vi "MultiChannelMES4HWSyncExample.vi"() -> ()   [LabVIEW 2025]
uses:
  PalmSens/PalmSens.lvclass
  PalmSens/MeasurementsResult.ctl
  PalmSens/MeasurementResults.ctl
  PalmSens/LiveCurveResult.ctl
  C:/Users/stef/code/palmsenssdk/labview/PalmSens/Libraries/PalmSens.Core.Simplified.LabVIEW.dll
  PalmSens/Libraries/PalmSens.Core.Simplified.LabVIEW.dll
panel:
  out "Array 2":string[](array[string])
  out "Is Measuring 2":bool
  in  "PalmSens.lvclass 2":refnum<class "PalmSens.lvclass">
  out "Measurements":T1
  out "MethodSCRIPT":refnum<k24>
  out "Array":string[](array[string])
  out "Is Measuring":bool
  in  "PalmSens.lvclass":refnum<class "PalmSens.lvclass">
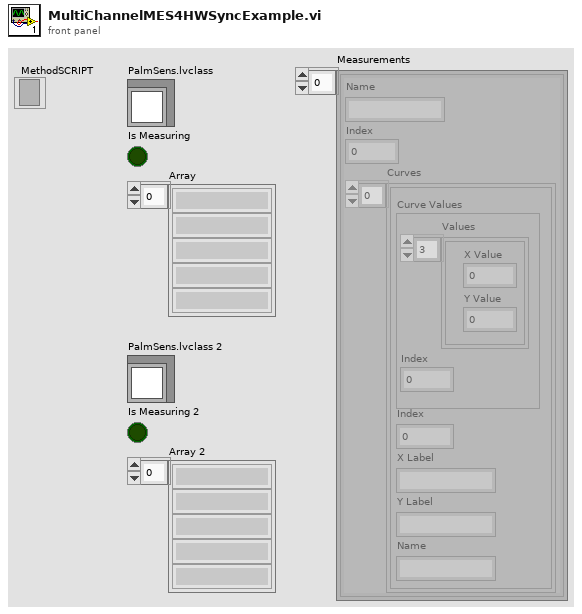
[diagram p1: front panel]
types:
  T1 = typedef "MeasurementsResult.ctl" = cluster{"Name":string, "Curves":T2, "Index":i32}[]
  T2 = typedef "MeasurementResults.ctl" = T3[]
  T3 = typedef "LiveCurveResult.ctl" = cluster{"X Label":string, "Y Label":string, "Name":string, "Index":i16, "Curve Values":cluster{"Values":cluster{"X Value":dbl, "Y Value":dbl}[], "Index":i16}}
  T4 = typedef "ActiveMeasurementInfo.ctl" = cluster{"Active Measurement":refnum<k24>, "Is Measuring Refnum":refnum<vi>, "Live Curve Result Refnum":refnum<vi>}
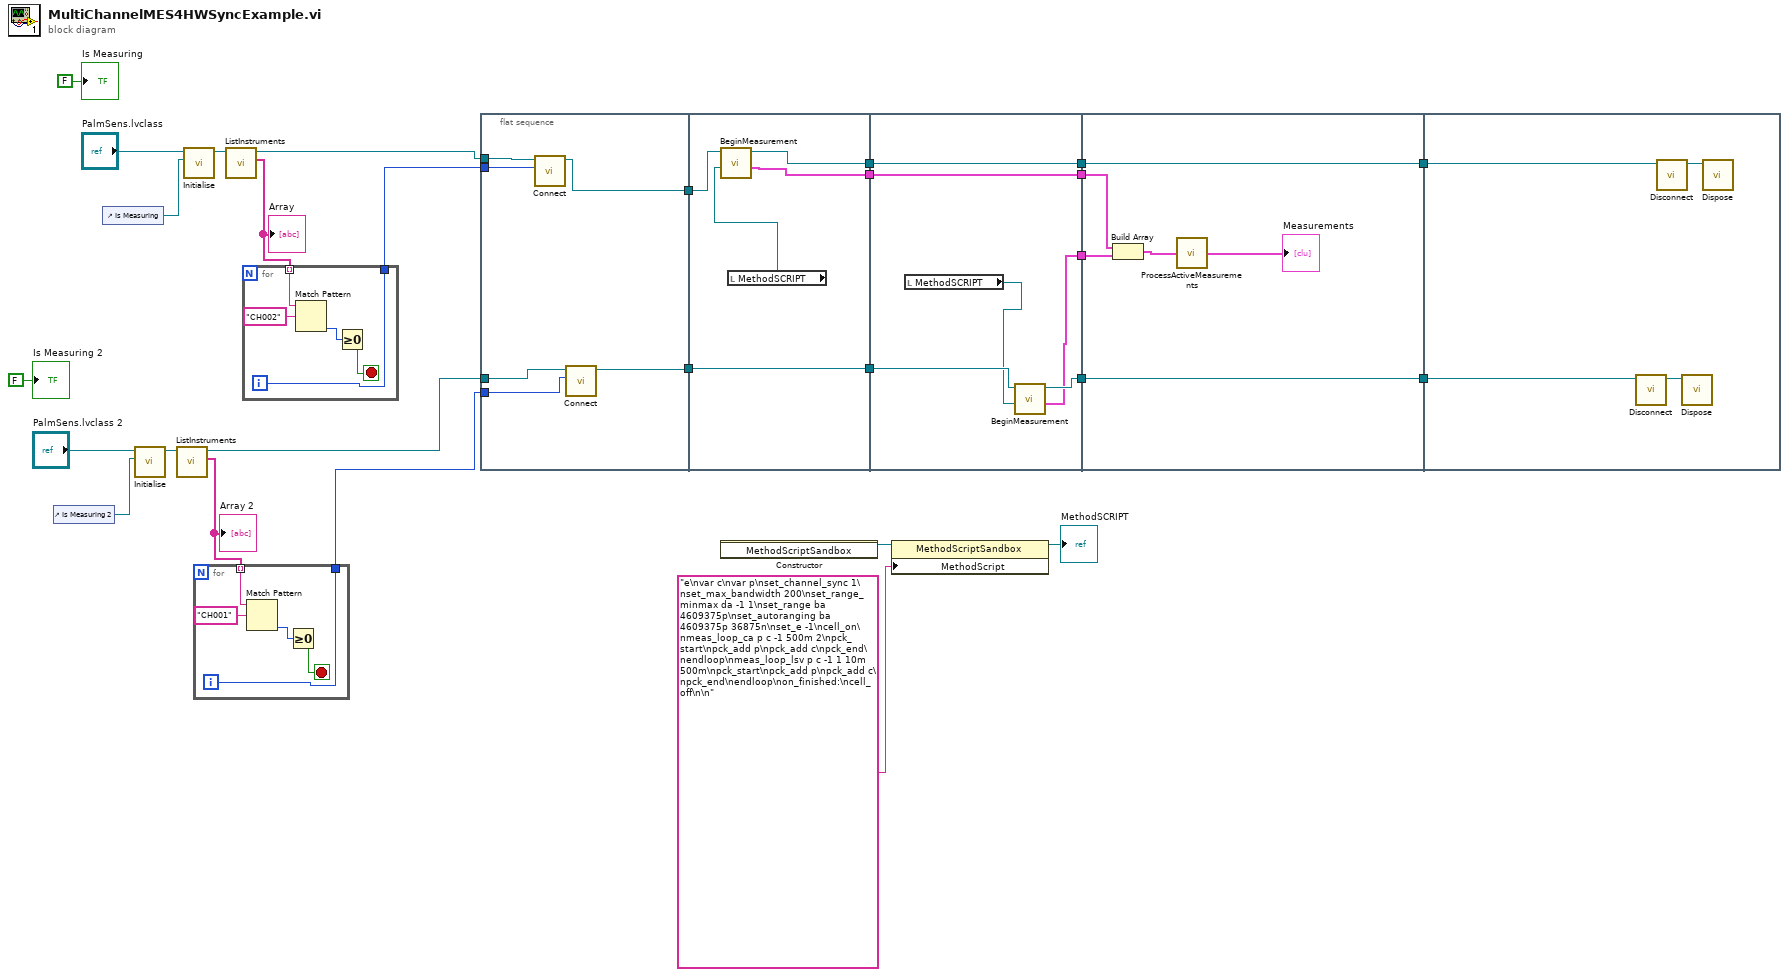
[diagram p0: block diagram]
diagram:
  n1 = control-ref of="Is Measuring 2"() -> (w7:refnum<vi>)
  n2 = control-ref of="Is Measuring"() -> (w27:refnum<vi>)
  n3 = call-dynamic "Initialise.vi"("Is Measuring Refnum"=w7, "PalmSens in"="PalmSens.lvclass 2") -> ("PalmSens out"=w6:refnum<class "PalmSens.lvclass">)  [unwired: 8 in, 1 out]
  n4 = call-dynamic "ListInstruments.vi"("PalmSens in"=w6) -> ("Array"=w5:string[], "PalmSens out"=w4:refnum<class "PalmSens.lvclass">)  [unwired: 8 in, 1 out]
  "Array 2" <- w5
  n5 = call-dynamic "Initialise.vi"("Is Measuring Refnum"=w27, "PalmSens in"="PalmSens.lvclass") -> ("PalmSens out"=w26:refnum<class "PalmSens.lvclass">)  [unwired: 8 in, 1 out]
  n6 = for {
    tunnel: w5 -> [w33] mode=indexing
    tunnel: [w29] -> w3
    i -> [w29]
    stop <- w32 stop-if-true
    n7 = Match Pattern(string=w33, regular expression="CH001") -> (offset past match=w31:i32)  [unwired: 1 in, 3 out]
    n8 = Greater Or Equal To 0?(x=w31) -> (x >= 0?=w32:bool)
  }
  n9 = call-dynamic "ListInstruments.vi"("PalmSens in"=w26) -> ("Array"=w22:string[], "PalmSens out"=w10:refnum<class "PalmSens.lvclass">)  [unwired: 8 in, 1 out]
  "Array" <- w22
  n10 = for {
    tunnel: w22 -> [w38] mode=indexing
    tunnel: [w34] -> w9
    i -> [w34]
    stop <- w37 stop-if-true
    n11 = Match Pattern(string=w38, regular expression="CH002") -> (offset past match=w36:i32)  [unwired: 1 in, 3 out]
    n12 = Greater Or Equal To 0?(x=w36) -> (x >= 0?=w37:bool)
  }
  n13 = flat-sequence {
    tunnel: [w42] -> w21
    tunnel: [w39] -> w20
    tunnel: w9 -> [w44]
    tunnel: w10 -> [w43]
    tunnel: w3 -> [w41]
    tunnel: w4 -> [w40]
    tunnel: [w47] -> w17
    tunnel: [w46] -> w14
    tunnel: w21 -> [w48]
    tunnel: w20 -> [w49]
    tunnel: [w49] -> w11
    tunnel: w17 -> [w55]
    tunnel: [w55] -> w16
    tunnel: [w52] -> w15
    tunnel: w14 -> [w54]
    tunnel: [w54] -> w13
    tunnel: [w51] -> w12
    tunnel: w11 -> [w53]
    tunnel: [w61] -> w19
    tunnel: [w60] -> w18
    tunnel: w16 -> [w61]
    tunnel: w15 -> [w60]
    tunnel: w13 -> [w59]
    tunnel: w12 -> [w58]
    tunnel: w19 -> [w63]
    tunnel: w18 -> [w62]
    frame #0 {
      n14 = call-dynamic "Connect.vi"("Instrument Index"=w44, "PalmSens in"=w43) -> ("PalmSens out"=w42:refnum<class "PalmSens.lvclass">)  [unwired: 8 in, 1 out]
      n15 = call-dynamic "Connect.vi"("Instrument Index"=w41, "PalmSens in"=w40) -> ("PalmSens out"=w39:refnum<class "PalmSens.lvclass">)  [unwired: 8 in, 1 out]
    }
    frame #1 {
      n16 = local read "MethodSCRIPT"() -> (w45:refnum<k24>)
      n17 = call-dynamic "BeginMeasurement.vi"("Method .NET Refnum"=w45, "PalmSens in"=w48) -> ("Active Measurement Info"=w46:T4, "PalmSens out"=w47:refnum<class "PalmSens.lvclass">)  [unwired: 2 in, 2 out]
    }
    frame #2 {
      n18 = local read "MethodSCRIPT"() -> (w50:refnum<k24>)
      n19 = call-dynamic "BeginMeasurement.vi"("Method .NET Refnum"=w50, "PalmSens in"=w53) -> ("Active Measurement Info"=w51:T4, "PalmSens out"=w52:refnum<class "PalmSens.lvclass">)  [unwired: 2 in, 2 out]
    }
    frame #3 {
      n20 = Build Array(w59, w58) -> (w57:T4[])
      n21 = call "ProcessActiveMeasurements.vi"("Active Measurements"=w57) -> ("Measurements"=→"Measurements":T1)
    }
    frame #4 {
      n22 = call-dynamic "Disconnect.vi"("PalmSens in"=w62) -> ("PalmSens out"=w64:refnum<class "PalmSens.lvclass">)  [unwired: 9 in, 1 out]
      n23 = call-dynamic "Disconnect.vi"("PalmSens in"=w63) -> ("PalmSens out"=w65:refnum<class "PalmSens.lvclass">)  [unwired: 9 in, 1 out]
      n24 = call-dynamic "Dispose.vi"("PalmSens in"=w64) -> ()  [unwired: 9 in, 2 out]
      n25 = call-dynamic "Dispose.vi"("PalmSens in"=w65) -> ()  [unwired: 9 in, 2 out]
    }
  }
  n26 = constructor class="MethodScriptSandbox"() -> (reference out=w25:refnum<k24>)  [unwired: 3 in, 2 out]
  n27 = property class="MethodScriptSandbox"(reference=w25, "MethodScript"="e\nvar c\nvar p\nset_channel_sync 1\nset_max_bandwidth 200\nset_range_minmax da -1 1\nset_range ba 4609375p\nset_autoranging ba 4609375p 36875n\nset_e -1\ncell_on\nmeas_loop_ca p c -1 500m 2\npck_start\npck_add p\npck_add c\npck_end\nendloop\nmeas_loop_lsv p c -1 1 10m 500m\npck_start\npck_add p\npck_add c\npck_end\nendloop\non_finished:\ncell_off\n\n") -> (reference out=→"MethodSCRIPT":refnum<k24>)  [unwired: 1 in, 1 out]
  "Is Measuring" <- FALSE ("Is Measuring")
  "Is Measuring 2" <- FALSE ("Is Measuring 2")
